vi "Find Air Pockets Connected to Exterior Surface.vi"(1 "Lava Droplets":set{cluster{"X":i32, "Y":i32, "Z":i32}}(c389), 2 "Z":i32[](array[numeric]), 3 "Y":i32[](array[numeric]), 4 "X":i32[](array[numeric])) -> (0 "Air Pockets Connected to Exterior Surface":set{cluster{"X":i32, "Y":i32, "Z":i32}}(c389))   [LabVIEW 2020, in "AoC 2022.lvlib"]
uses:
  AoC 2022.lvlib
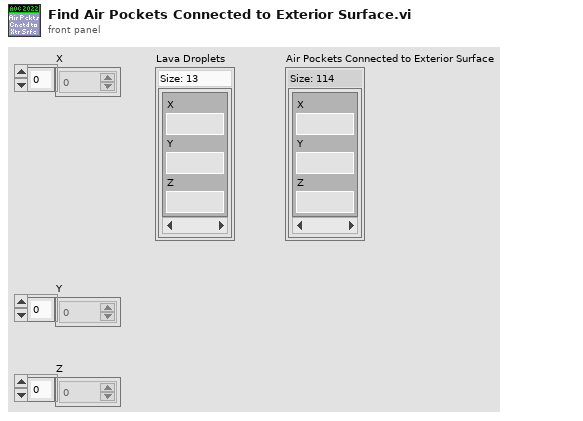
[diagram p1: front panel]
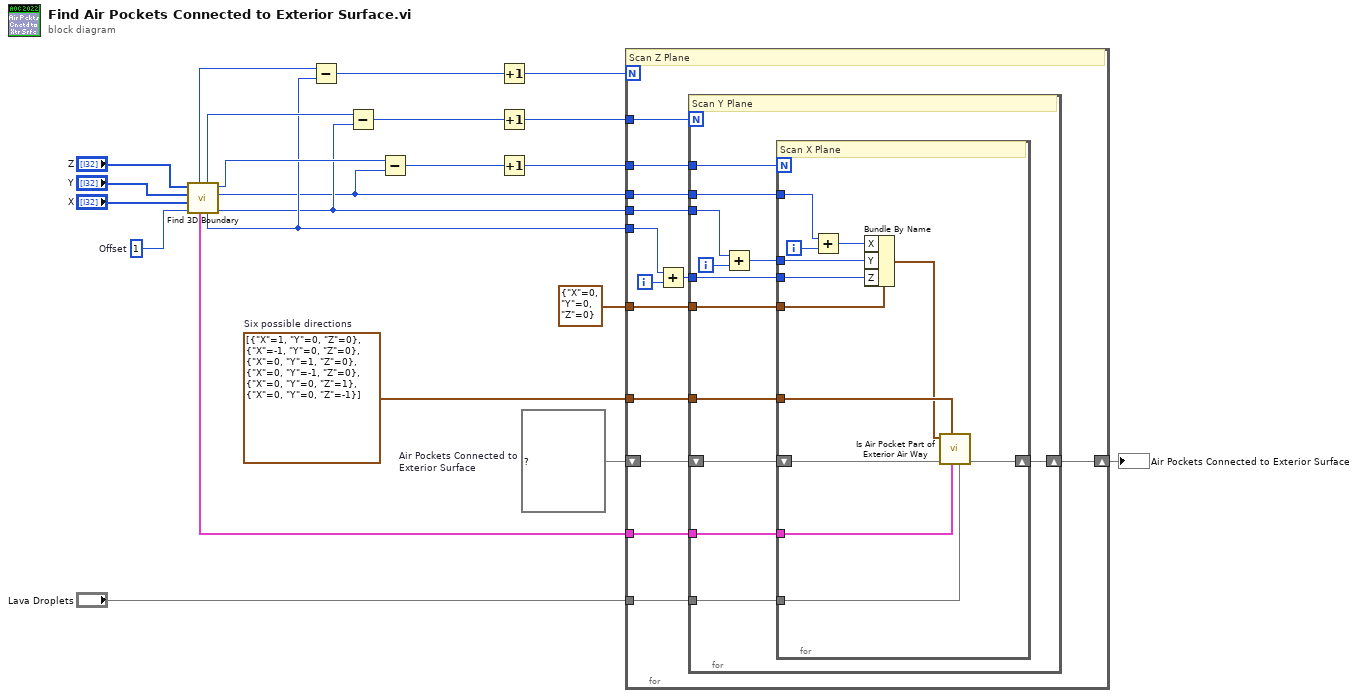
[diagram p0: block diagram]
diagram:
  w11 = 1  # Offset
  w21 = set{cluster{"X":i32, "Y":i32, "Z":i32}} {}  # Air Pockets Connected to Exterior Surface
  w18 = cluster{"X":i32, "Y":i32, "Z":i32}[] [{"X"=1, "Y"=0, "Z"=0}, {"X"=-1, "Y"=0, "Z"=0}, {"X"=0, "Y"=1, "Z"=0}, {"X"=0, "Y"=-1, "Z"=0}, {"X"=0, "Y"=0, "Z"=1}, {"X"=0, "Y"=0, "Z"=-1}]  # Six possible directions
  n1 = call "Find 3D Boundary.vi"("Offset"=w11, "X"="X", "Y"="Y", "Z"="Z") -> ("Y Min"=w5:i32, "X Min"=w4:i32, "X Max"=w14:i32, "Z Min"=w9:i32, "Y Max"=w15:i32, "Extreme Planes"=w12:cluster{"X":i32[], "Y":i32[], "Z":i32[]}, "Z Max"=w10:i32)  [unwired: 1 in]
  n2 = Subtract(x=w10, y=w9) -> (x-y=w8:i32)
  n3 = Subtract(x=w15, y=w5) -> (x-y=w7:i32)
  n4 = Subtract(x=w14, y=w4) -> (x-y=w6:i32)
  n5 = Increment(x=w8) -> (x+1=w1:i32)
  n6 = Increment(x=w7) -> (x+1=w2:i32)
  n7 = Increment(x=w6) -> (x+1=w3:i32)
  n8 = for {
    N: w1 -> [_]
    tunnel: w2 -> [w34]
    tunnel: w5 -> [w33]
    tunnel: w3 -> [w32]
    tunnel: w4 -> [w31]
    tunnel: cluster{"X":i32, "Y":i32, "Z":i32} {"X"=0, "Y"=0, "Z"=0} -> [w30]
    shift-right: [w27] -> w16
    shift-left: w21 -> [w28]
    tunnel: w18 -> [w26]
    tunnel: "Lava Droplets" -> [w25]
    tunnel: w12 -> [w23]
    tunnel: w9 -> [w24]
    i -> [w35]
    # "Scan Z Plane"
    n9 = Add(x=w24, y=w35) -> (x+y=w29:i32)
    n10 = for {
      N: w34 -> [_]
      tunnel: w33 -> [w47]
      tunnel: w32 -> [w45]
      tunnel: w31 -> [w44]
      tunnel: w30 -> [w43]
      tunnel: w29 -> [w42]
      shift-right: [w39] -> w27
      shift-left: w28 -> [w40]
      tunnel: w26 -> [w38]
      tunnel: w25 -> [w37]
      tunnel: w23 -> [w36]
      i -> [w46]
      # "Scan Y Plane"
      n11 = Add(x=w47, y=w46) -> (x+y=w41:i32)
      n12 = for {
        N: w45 -> [_]
        tunnel: w44 -> [w58]
        tunnel: w43 -> [w57]
        tunnel: w42 -> [w56]
        tunnel: w41 -> [w55]
        shift-right: [w53] -> w39
        shift-left: w40 -> [w48]
        tunnel: w38 -> [w52]
        tunnel: w37 -> [w51]
        tunnel: w36 -> [w49]
        i -> [w59]
        # "Scan X Plane"
        n13 = Add(x=w58, y=w59) -> (x+y=w54:i32)
        n14 = Bundle By Name(cluster=w57, "X"=w54, "Y"=w55, "Z"=w56) -> (w50:cluster{"X":i32, "Y":i32, "Z":i32})
        n15 = call "Is Air Pocket Part of Exterior Air Way.vi"("Lava Droplets"=w51, "Extreme Planes"=w49, "Possible Directions"=w52, "Air Pockets Connected to Exterior Surface in"=w48, "Location"=w50) -> ("Air Pockets Connected to Exterior Surface out"=w53:set{cluster{"X":i32, "Y":i32, "Z":i32}})  [unwired: 3 in, 2 out]
      }
    }
  }
  "Air Pockets Connected to Exterior Surface" <- w16
